vi "EG_G5210 ParString.vi"(8 "entrée d'erreur (pas d'erreur)":errorcluster, 11 "LockInPar":T1={"Sensitivity"=1, "Vernier Mode"=FALSE, "Vernier Value"=0, "Main Filter"=0, "Filter Freq (Hz)"=0.0, "Filter Mode"=0, " Line Notch"=0, "Reference"=0, "Reference Mode"=0, "Ref Phase (°)"=0.0, "Ref Freq (Hz)"=0.0, "Output Filter"=0, "Time Constant"=1, "Dynamic Res."=0, "X Offset"=FALSE, "X Offset Val %"=0.0, "Y Offset"=FALSE, "Y Offset Val %"=0.0, "Expand"=FALSE, "Int Osc (Vrms)"=0.0, "Int Osc (Hz)"=0.0, "Trigger Mode"=0, "Input Mode"=0, "Ovld Source"=0} caption="Lock-In Parameters" {"Ovld Source" items=["Y Channel", "X Channel", "PSD", "Input", "Ref Unlck"]; "Input Mode" items=["Current 10E8 A/V", "Current 10E6 A/V", "Voltage"]; "Trigger Mode" items=["Reference", "External", "Asynchronous", "Ratio", "8F"]; "Reference Mode" items=["F", "2F"]; "Reference" items=["External", "Internal"]; "Filter Mode" items=["Manual", "Automatic"]; "Line Notch" items=["Off", "120 Hz", "60 Hz", "Both"]; "Main Filter" items=["No Filter", "Notch", "Low Pass", "Band Pass"]; "Output Filter" items=["6dB", "12dB"]; "Time Constant" items=["1 ms", "3 ms", "10 ms", "30 ms", "100 ms", "300 ms", "1 s", "3 s", "10 s", "30 s", "100 s", "300 s", "1000 s", "3000 s"]; "Sensitivity" items=["100 nV", "300 nV", "1 µV", "3 µV", "10 µV", "30 µV", "100µV", "300 µV", "1 mV", "3 mV", "10 mV", "30 mV", "100 mV", "300 mV", "1 V", "3 V"]; "Dynamic Res." items=["Hi Stab", "Normal", "Hi Res"]}) -> (0 "sortie d'erreur":errorcluster, 3 "Chaîne":string)   [LabVIEW 2010]
uses:
  <userlib>/EG_G 5210 LIA/LockInPar.ctl
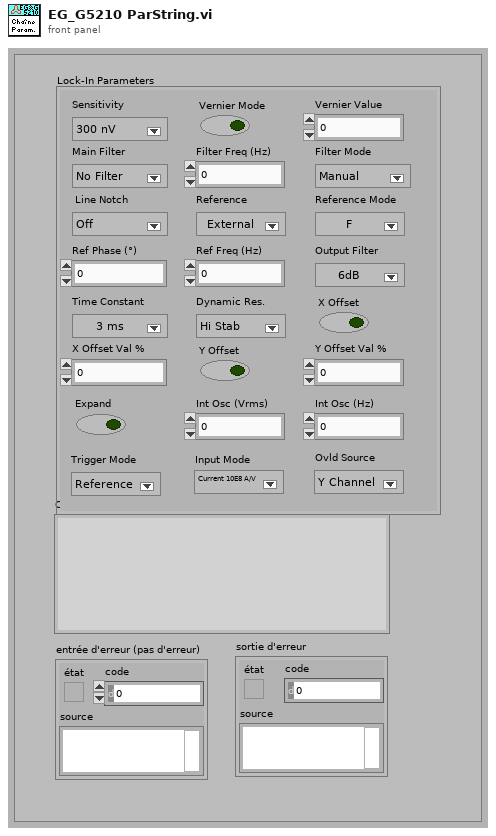
[diagram p1: front panel]
types:
  T1 = typedef "LockInPar.ctl" = cluster{"Sensitivity":u16, "Vernier Mode":bool, "Vernier Value":i32, "Main Filter":u16, "Filter Freq (Hz)":dbl, "Filter Mode":u16, " Line Notch":u16, "Reference":u16, "Reference Mode":u16, "Ref Phase (°)":dbl, "Ref Freq (Hz)":dbl, "Output Filter":u16, "Time Constant":u16, "Dynamic Res.":u16, "X Offset":bool, "X Offset Val %":dbl, "Y Offset":bool, "Y Offset Val %":dbl, "Expand":bool, "Int Osc (Vrms)":dbl, "Int Osc (Hz)":dbl, "Trigger Mode":u16, "Input Mode":u16, "Ovld Source":u16}
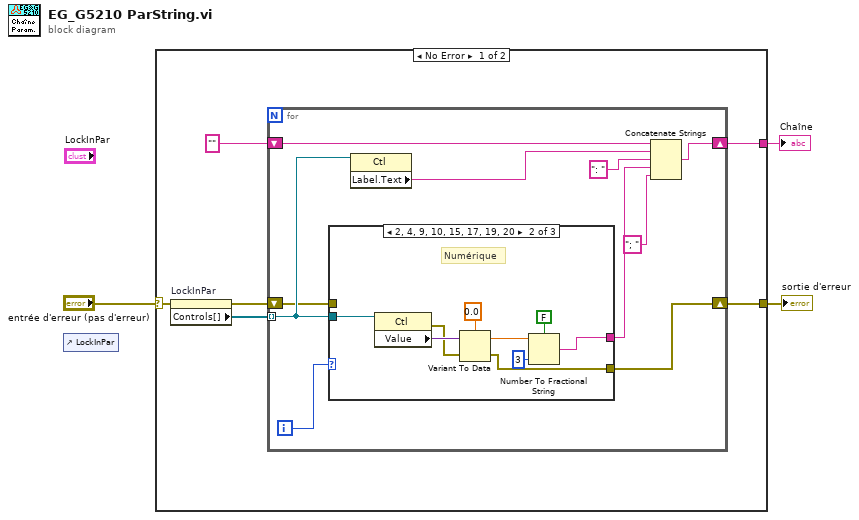
[diagram p0: block diagram]
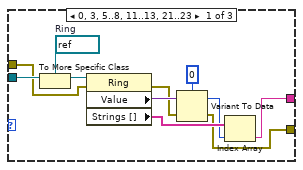
[diagram p2: hidden frame]
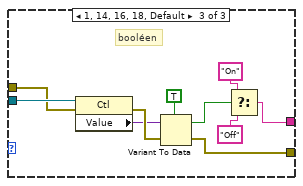
[diagram p3: hidden frame]
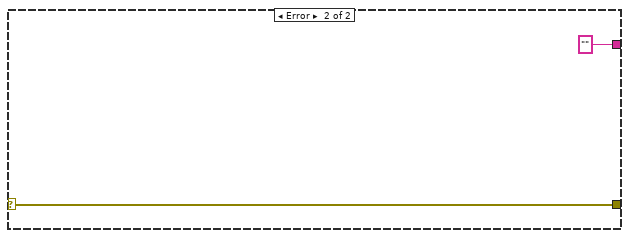
[diagram p4: hidden frame]
diagram:
  n1 = control-ref of="LockInPar"() -> ()  [unwired: 1 out]
  n2 = case shown="No Error" "entrée d'erreur (pas d'erreur)" {
    selector: "entrée d'erreur (pas d'erreur)" -> [w6 w51]
    tunnel: [w8 ""] -> w3
    tunnel: [w7 w51] -> w2
    frame No Error {
      n3 = property on="LockInPar" class="Clust (strict)"(error in=w6) -> (error out=w4:errorcluster, "Controls[]"=w5:refnum<vi>[])  [unwired: 1 in, 1 out]
      n4 = for {
        tunnel: w5 -> [w18] mode=indexing
        shift-right: [w14] -> w8
        shift-left: "" -> [w13]
        shift-right: [w10] -> w7
        shift-left: w4 -> [w11]
        i -> [w19]
        n5 = case shown="2, 4, 9, 10, 15, 17, 19, 20" w19 {
          tunnel: [w26 w35 w43] -> w15
          tunnel: w18 -> [w25 w34 w42]
          tunnel: w11 -> [w21 _ w41]
          tunnel: [w20 w33 w40] -> w10
          frame 0, 3, 5..8, 11..13, 21..23 {
            w24 = refnum<vi> refnum  # Ring
            n6 = To More Specific Class(target class=w24, reference=w25) -> (specific class reference=w23:refnum<vi>)  [unwired: 1 in, 1 out]
            n7 = property class="Ring"(reference=w23, error in=w21) -> (error out=w27:errorcluster, "Value"=w28:variant, "Strings []"=w30:string[])  [unwired: 1 out]
            n8 = Variant To Data(error in=w27, Variant=w28, type=0) -> (error out=w20:errorcluster, data=w22:i32)
            n9 = Index Array(array=w30, index=w22) -> (element=w26:string)
          }
          frame 2, 4, 9, 10, 15, 17, 19, 20 {
            # "Numérique"
            n10 = property class="Ctl"(reference=w34) -> (error out=w38:errorcluster, "Value"=w39:variant)  [unwired: 1 in, 1 out]
            n11 = Variant To Data(error in=w38, Variant=w39, type=0.0) -> (error out=w33:errorcluster, data=w36:dbl)
            n12 = Number To Fractional String(use system decimal point (T)=FALSE ("utiliser le séparateur décimal du système (V)"), number=w36, precision (6)=i16 3 ("précision (6)")) -> (F-format string=w35:string)  [unwired: 1 in]
          }
          frame 1, 14, 16, 18, Default {
            # "booléen"
            n13 = property class="Ctl"(reference=w42, error in=w41) -> (error out=w49:errorcluster, "Value"=w48:variant)  [unwired: 1 out]
            n14 = Variant To Data(error in=w49, Variant=w48, type=TRUE) -> (error out=w40:errorcluster, data=w46:bool)
            n15 = Select(t="On", s=w46, f="Off") -> (s? t:f=w43:string)
          }
        }
        n16 = property class="Ctl"(reference=w18) -> ("Label.Text"=w17:string)  [unwired: 1 in, 2 out]
        n17 = Concatenate Strings(w13, w17, ": " ("chaîne"), w15, "; " ("chaîne")) -> (w14:string)
      }
    }
    frame Error {
    }
  }
  "Chaîne" <- w3
  "sortie d'erreur" <- w2
